vi "cDAQ DDS Config Panel.vi"(8 "error in":errorcluster, 11 "cDAQ dds":T3={"device"="", "channels"=[], "mclk source"="", "mclk [Hz]"=0.0, "fs [Hz]"=0.0, "block [s]"=0.0, "buf [s]"=0.0, "task"="", "cmd queue"=refnum, "proc ref"=refnum, "smpl clock out"="/cDAQ3/PFI0", "export smpl clock"=FALSE, "DC ofs [V]"=[], "timebase source"="", "timebase mode"=enum."Local", "dither"=enum."Disabled", "dither level"=0.0} {"channels" min=0 step=1}) -> (0 "error out":errorcluster, 3 "cDAQ dds out":T3={"device"="", "channels"=[], "mclk source"="", "mclk [Hz]"=0.0, "fs [Hz]"=0.0, "block [s]"=0.0, "buf [s]"=0.0, "task"="", "cmd queue"=refnum, "proc ref"=refnum, "smpl clock out"="/cDAQ3/PFI0", "export smpl clock"=FALSE, "DC ofs [V]"=[], "timebase source"="", "timebase mode"=enum."Local", "dither"=enum."Disabled", "dither level"=0.0} {"channels" min=0 step=1})   [LabVIEW 2020]
uses:
  cDAQ DDS Session.ctl
  cDAQ DDS Setup.ctl
  cDAQ DDS Timebase Mode.ctl
  cDAQ DDS Dither.ctl
panel:
  in  "dither level":dbl caption="Dithering level [V]" format="%#_6p"
  in  "dither":T1 caption="Dithering mode"
  in  "timebase mode":T2 caption="Timebase mode"
  in  "btn default":bool caption="OK Button"
  in  "timebase src":tag caption="Timebase source"
  in  "DC offset [V]":dbl[](array[numeric])
  in  "smpl clock dest":tag="/cDAQ3/PFI0" caption="Sample clock destination"
  in  "export smpl clk":bool caption="Export sample clock"
  in  "btn test":bool caption="OK Button"
  in  "chn idx":i32[](array[numeric]) caption="Channel indices"
  in  "btn ok":bool caption="OK Button"
  in  "dac fs":dbl=50000.0 caption="DAC sampling rate [Sa/s]" format="%#_6p"
  in  "block [s]":dbl=0.2 caption="Write block size [s]"
  in  "buf size [s]":dbl=1.0 caption="DAC buffer size [s]"
  in  "mckl freq [Hz]":dbl=12800000.0 caption="Reference timebase frequency [Hz]" format="%#_6p"
  in  "mckl device":tag caption="Reference clock device address"
  in  "device":tag caption="DAC device address"
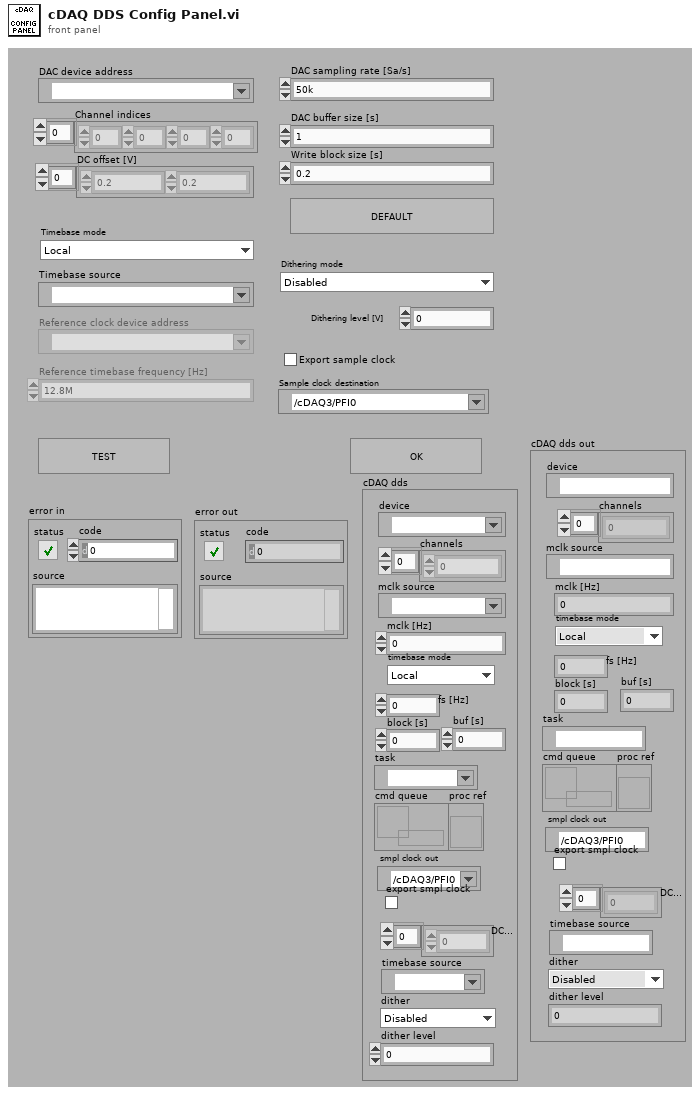
[diagram p1: front panel]
types:
  T1 = typedef "cDAQ DDS Dither.ctl" = enum16{"Disabled", "Gaussian"}
  T2 = typedef "cDAQ DDS Timebase Mode.ctl" = enum16{"Local", "Take from ADC (e.g. NI 9238)", "Other source"}
  T3 = typedef "cDAQ DDS Session.ctl" = cluster{"device":tag, "channels":i32[], "mclk source":tag, "mclk [Hz]":dbl, "fs [Hz]":dbl, "block [s]":dbl, "buf [s]":dbl, "task":refnum<k21>, "cmd queue":refnum<queue>, "proc ref":refnum<vi>, "smpl clock out":tag, "export smpl clock":bool, "DC ofs [V]":dbl[], "timebase source":tag, "timebase mode":T2, "dither":T1, "dither level":dbl}
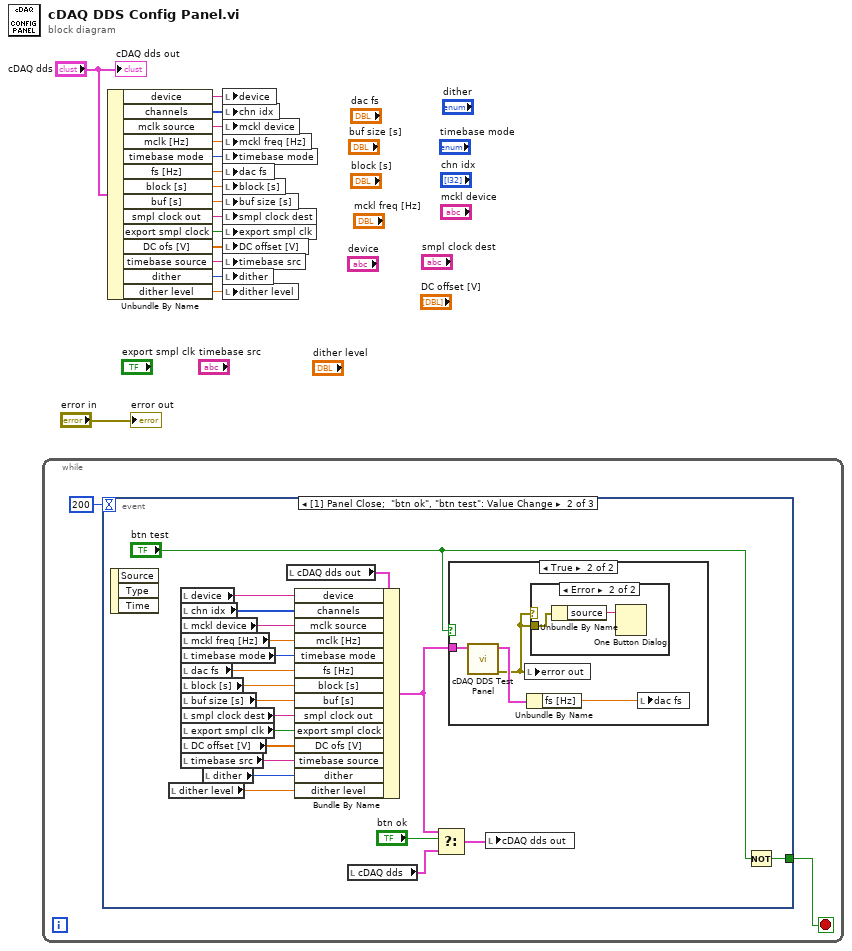
[diagram p0: block diagram]
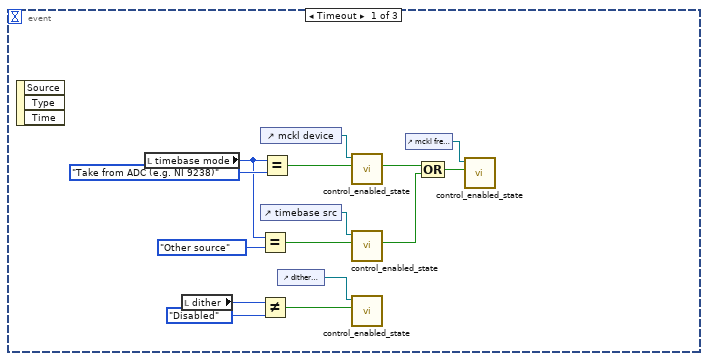
[diagram p2: hidden frame]
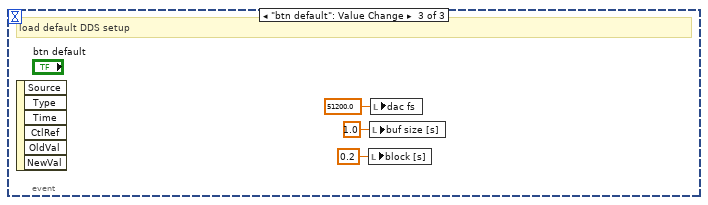
[diagram p5: hidden frame]
diagram:
  n1 = while {
    stop <- w18 stop-if-true
    n2 = event shown="[1] Panel Close;  \"btn ok\", \"btn test\": Value Change" {
      selector: _ -> [_ _ _]
      dyn-events: _ -> [_ _ _]
      timeout: 200 -> [_ _ _]
      tunnel: [_ w42 _] -> w18
      event Timeout {
        n3 = event-data() -> ()  [unwired: 1 in, 3 out]
        n4 = local read "timebase mode"() -> (w27:T2)
        n5 = local read "dither"() -> (w20:T1)
        n6 = Equal?(x=w27, y=cDAQ_DDS_Timebase_Mode."Other source") -> (x = y?=w29:bool)
        n7 = Not Equal?(x=w20, y=cDAQ_DDS_Dither."Disabled") -> (x != y?=w21:bool)
        n8 = control-ref of="mckl device"() -> (w33:refnum<vi>)
        n9 = control-ref of="timebase src"() -> (w28:refnum<vi>)
        n10 = Equal?(x=w27, y=cDAQ_DDS_Timebase_Mode."Take from ADC (e.g. NI 9238)") -> (x = y?=w30:bool)
        n11 = control-ref of="dither level"() -> (w22:refnum<vi>)
        n12 = call "control_enabled_state.vi"("enabled"=w30, "control in"=w33) -> ("enabled"=w25:bool)  [unwired: 6 in, 3 out]
        n13 = call "control_enabled_state.vi"("enabled"=w29, "control in"=w28) -> ("enabled"=w24:bool)  [unwired: 6 in, 3 out]
        n14 = call "control_enabled_state.vi"("enabled"=w21, "control in"=w22) -> ()  [unwired: 6 in, 4 out]
        n15 = control-ref of="mckl freq [Hz]"() -> (w32:refnum<vi>)
        n16 = Compound Arithmetic op=OR(w25, w24) -> (w23:bool)
        n17 = call "control_enabled_state.vi"("enabled"=w23, "control in"=w32) -> ()  [unwired: 6 in, 4 out]
      }
      event Panel Close; "btn ok", "btn test": Value Change {
        n18 = event-data() -> ()  [unwired: 1 in, 3 out]
        n19 = local read "dither level"() -> (w34:dbl)
        n20 = local read "device"() -> (w51:tag)
        n21 = local read "chn idx"() -> (w50:i32[])
        n22 = local read "mckl device"() -> (w49:tag)
        n23 = local read "mckl freq [Hz]"() -> (w48:dbl)
        n24 = local read "timebase mode"() -> (w47:T2)
        n25 = local read "dac fs"() -> (w46:dbl)
        n26 = local read "block [s]"() -> (w45:dbl)
        n27 = local read "buf size [s]"() -> (w44:dbl)
        n28 = local read "smpl clock dest"() -> (w39:tag)
        n29 = local read "export smpl clk"() -> (w38:bool)
        n30 = local read "DC offset [V]"() -> (w37:dbl[])
        n31 = local read "timebase src"() -> (w36:tag)
        n32 = local read "dither"() -> (w35:T1)
        n33 = local read "cDAQ dds out"() -> (w52:T3)
        n34 = Bundle By Name(cluster=w52, "device"=w51, "channels"=w50, "mclk source"=w49, "mclk [Hz]"=w48, "timebase mode"=w47, "fs [Hz]"=w46, "block [s]"=w45, "buf [s]"=w44, "smpl clock out"=w39, "export smpl clock"=w38, "DC ofs [V]"=w37, "timebase source"=w36, "dither"=w35, "dither level"=w34) -> (w41:T3)
        n35 = local read "cDAQ dds"() -> (w54:T3)
        n36 = Select(t=w41, s="btn ok", f=w54) -> (s? t:f=w53:T3)
        n37 = case shown="True" "btn test" {
          tunnel: w41 -> [_ w58]
          frame False {
          }
          frame True {
            n38 = call "cDAQ DDS Test Panel.vi"("cDAQ dds"=w58) -> ("error out"=w55:errorcluster, "cDAQ dds out"=w57:T3)  [unwired: 9 in]
            n39 = local write "error out"(w55) -> ()
            n40 = Unbundle By Name(w57) -> ("fs [Hz]"=w56:dbl)
            n41 = case shown="Error" w55 {
              tunnel: w55 -> [_ w59]
              frame No Error {
              }
              frame Error {
                n42 = Unbundle By Name(w59) -> ("source"=w60:string)
                n43 = One Button Dialog(message=w60) -> ()  [unwired: 1 in, 1 out]
              }
            }
            n44 = local write "dac fs"(w56) -> ()
          }
        }
        n45 = local write "cDAQ dds out"(w53) -> ()
        n46 = Not(x="btn test") -> (.not. x?=w42:bool)
      }
      event "btn default": Value Change {
        # "load default DDS setup"
        n47 = event-data() -> ()  [unwired: 1 in, 6 out]
        n48 = local write "block [s]"(0.2 ("block [s]")) -> ()
        n49 = local write "buf size [s]"(1.0 ("buf size [s]")) -> ()
        n50 = local write "dac fs"(51200.0 ("dac fs")) -> ()
      }
    }
  }
  n51 = Unbundle By Name("cDAQ dds") -> ("device"=w15:tag, "channels"=w14:i32[], "mclk source"=w13:tag, "mclk [Hz]"=w12:dbl, "timebase mode"=w11:T2, "fs [Hz]"=w10:dbl, "block [s]"=w9:dbl, "buf [s]"=w8:dbl, "smpl clock out"=w6:tag, "export smpl clock"=w5:bool, "DC ofs [V]"=w4:dbl[], "timebase source"=w3:tag, "dither"=w2:T1, "dither level"=w1:dbl)
  n52 = local write "device"(w15) -> ()
  n53 = local write "chn idx"(w14) -> ()
  n54 = local write "mckl device"(w13) -> ()
  n55 = local write "mckl freq [Hz]"(w12) -> ()
  n56 = local write "timebase mode"(w11) -> ()
  n57 = local write "dac fs"(w10) -> ()
  n58 = local write "block [s]"(w9) -> ()
  n59 = local write "buf size [s]"(w8) -> ()
  n60 = local write "smpl clock dest"(w6) -> ()
  n61 = local write "export smpl clk"(w5) -> ()
  n62 = local write "DC offset [V]"(w4) -> ()
  n63 = local write "timebase src"(w3) -> ()
  n64 = local write "dither"(w2) -> ()
  n65 = local write "dither level"(w1) -> ()
  "error out" <- "error in"
  "cDAQ dds out" <- "cDAQ dds"
